vi "Device State Information Update.vi"(8 "error in":errorcluster, 10 "Device State Information":T1={"Device State"=enum."DevIDs in Config", "data"=variant}, 11 "EMS User Interface in":refnum<class "EMS User Interface.lvclass">) -> (0 "error out":errorcluster, 3 "dup EMS User Interface":refnum<class "EMS User Interface.lvclass">)   [LabVIEW 2018, in "EMS User Interface Actor.lvlib" / "EMS User Interface.lvclass"]
uses:
  EMS User Interface.lvclass
  EMS Generic Actor/EMS Generic/Controls/Device Information Cluster.ctl
  EMS Generic Actor/EMS Generic/Controls/Device State.ctl
  EMS User Interface.lvclass/EMS User Interface.ctl
  EMS Generic Actor/EMS Generic/EMS Generic.lvclass
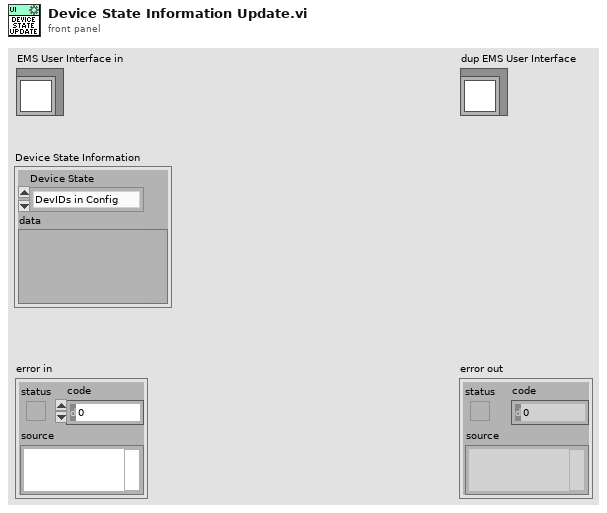
[diagram p1: front panel]
types:
  T1 = typedef "EMS Generic Actor.lvlib/EMS Generic.lvclass/Device Information Cluster.ctl" = cluster{"Device State":T2, "data":variant}
  T2 = typedef "EMS Generic Actor.lvlib/EMS Generic.lvclass/Device State.ctl" = enum16{"Invalid", "Clear", "DevIDs in Config", "DevIDs on uGrid", "DevIDs not on uGrid", "Update IED_Status", "Update DER_Status", "Update DER_Measurement", "Update SmartRelay_Measurement"}
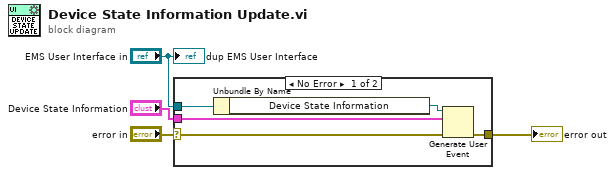
[diagram p0: block diagram]
diagram:
  n1 = case shown="No Error" "error in" {
    selector: "error in" -> [w6 w10]
    tunnel: [w5 w10] -> w3
    tunnel: "EMS User Interface in" -> [w8 _]
    tunnel: "Device State Information" -> [w9 _]
    frame No Error {
      n2 = Unbundle By Name(w8) -> ("Device State Information"=w7:refnum<user-event>)
      n3 = Generate User Event(user event=w7, event data cluster=w9, error in=w6) -> (error out=w5:errorcluster)  [unwired: 1 in, 1 out]
    }
    frame Error {
    }
  }
  "error out" <- w3
  "dup EMS User Interface" <- "EMS User Interface in"
